vi "BRig_dataCurrent_DAB_I_giveReward_R.vi"() -> (2 "output_DAB_I_giveReward_R":i32)   [LabVIEW 2014]
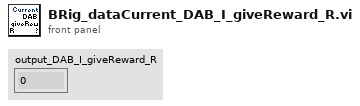
[diagram p1: front panel]
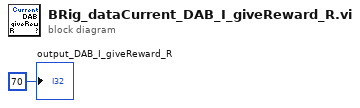
[diagram p0: block diagram]
diagram:
  "output_DAB_I_giveReward_R" <- 70 ("output_iBlock")
